vi "EXTToI64.vi"(5 "Number":ext) -> (1 "Signed 64-bit integer":i64, 2 "Overflow?":bool, 3 "Exact conversion?":bool)   [LabVIEW 2017, in "GPOverflow.lvlib"]
doc: "Converts <B>Number</B> to I64 keeping track of numeric overflow and exactness of conversion.\n\n<B>Exact conversion?</B> will be True only if a conversion back into the original data type of <B>Number</B> will yield the exact same number, i.e. no precision was lost during the conversion.\n\n<B>Overflow?</B> will be True if positive or negative overflow occurred. The numeric output will saturate in case of overflow.\n\nThis VI is inlined.\n\nSteen Schmidt\nGPower\n9/3 2013"
uses:
  GPOverflow.lvlib
  Comparison/GPComparison.lvlib
  Comparison/Library/IsInt/IsIntEXT.vi
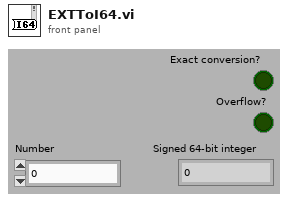
[diagram p1: front panel]
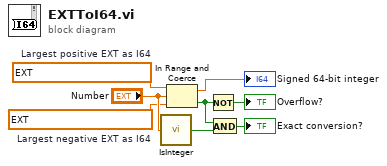
[diagram p0: block diagram]
diagram:
  w1 = ext -9223372036854775807.0  # Largest negative EXT as I64
  w2 = ext 9223372036854775807.0  # Largest positive EXT as I64
  n1 = call-poly "IsInteger.vi"("x"="Number") -> ("Integer?"=w6:bool)  [unwired: 4 in]
  n2 = In Range and Coerce(upper limit=w2, x="Number", lower limit=w1) -> (coerced(x)=→"Signed 64-bit integer":ext, In Range?=w4:bool)
  n3 = Not(x=w4) -> (.not. x?=→"Overflow?":bool)
  n4 = And(x=w4, y=w6) -> (x .and. y?=→"Exact conversion?":bool)
